vi "TS Results Base Path Create.vi"(8 "error in":errorcluster, 11 "Generic Test Stand in":refnum<class "Generic Test Stand.lvclass">) -> (0 "error out":errorcluster, 3 "Generic Test Stand out":refnum<class "Generic Test Stand.lvclass">)   [LabVIEW 2019, in "Generic Test Stand.lvclass"]
uses:
  Generic Test Stand.lvclass
  Generic Test Stand.lvclass/Generic Test Stand.ctl
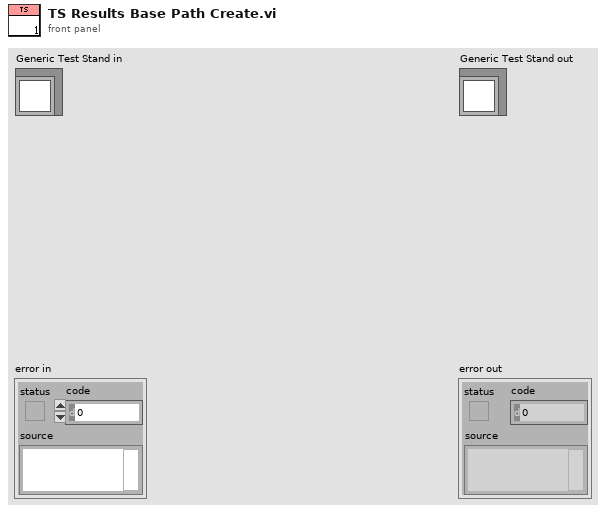
[diagram p1: front panel]
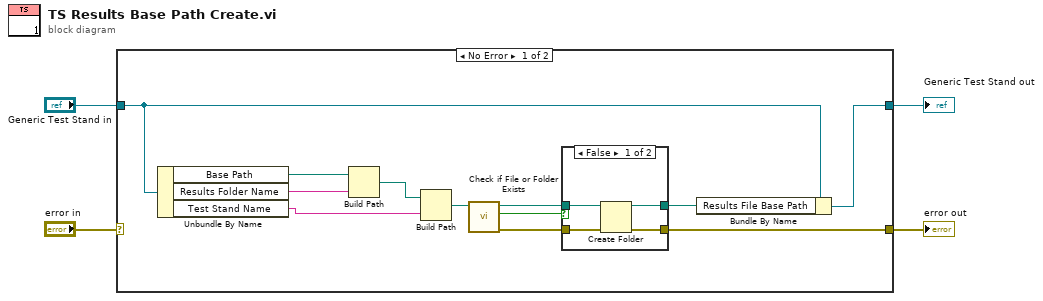
[diagram p0: block diagram]
diagram:
  n1 = case shown="No Error" "error in" {
    selector: "error in" -> [_ w24]
    tunnel: [w7 w24] -> w2
    tunnel: "Generic Test Stand in" -> [w10 w23]
    tunnel: [w8 w23] -> w1
    frame No Error {
      n2 = Unbundle By Name(w10) -> ("Base Path"=w11:path, "Results Folder Name"=w6:string, "Test Stand Name"=w5:string)
      n3 = Build Path(base path=w11, name or relative path=w6) -> (appended path=w13:path)
      n4 = Build Path(base path=w13, name or relative path=w5) -> (appended path=w12:path)
      n5 = call <vilib>:"Check if File or Folder Exists.vi"("path"=w12) -> ("error out"=w14:errorcluster, "file or folder exists?"=w16:bool, "dup path"=w15:path)  [unwired: 8 in]
      n6 = case shown="False" w16 {
        tunnel: w15 -> [w20 w22]
        tunnel: w14 -> [w19 w21]
        tunnel: [w17 w22] -> w9
        tunnel: [w18 w21] -> w7
        frame False {
          n7 = Create Folder(path (use dialog)=w20, error in=w19) -> (created path=w17:path, error out=w18:errorcluster)  [unwired: 1 in, 1 out]
        }
        frame True {
        }
      }
      n8 = Bundle By Name(cluster=w10, "Results File Base Path"=w9) -> (w8:refnum<class "Generic Test Stand.lvclass">)
    }
    frame Error {
    }
  }
  "error out" <- w2
  "Generic Test Stand out" <- w1
